vi "Drive_Heading.vi"(1 "Timeout (ms)":dbl, 2 "Speed (%)":dbl, 3 "Acceptable Error (in)":dbl, 4 "Distance (in)":dbl) -> (0 "Error (in)":dbl)   [LabVIEW 2020]
uses:
  <vilib>/Rock Robotics/WPI/ThirdParty/REV Robotics/REVLib/Typedef/Spark MAX Control Type.ctl
  <vilib>/Rock Robotics/WPI/ThirdParty/Phoenix-LabVIEW/Pigeon IMU/CTRE_PigeonIMU_GetYPR.vi
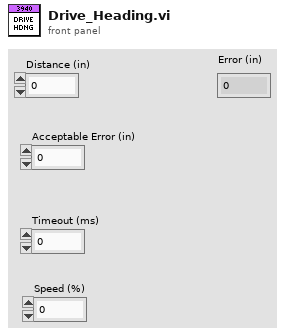
[diagram p1: front panel]
types:
  T1 = typedef "Spark MAX Control Type.ctl" = enum16{"Percent VBus", "Voltage", "Velocity", "Position", "Smart Motion", "Current", "Smart Velocity"}
  T2 = typedef "WPI_MotorControlDeviceRef.ctl" = cluster{"DeviceStatus":errorcluster, "Type":T3, "PWM":cluster{"PWM Channel":T4, "DeadBand":T5}, "CAN":cluster{"Device Number":u8, "SetOutput VI Ref":variant, "GetOutput VI Ref":variant, "Enable VI Ref":variant, "Disable VI Ref":variant, "Data":variant}, "Invert":bool, "DIO PWM":cluster{"PWM \"Enable\" Channel":T4, "DIOChannel":T6, "PWM Rate":dbl}}
  T3 = typedef "WPI_MotorControlType.ctl" = enum16{"PWM", "CAN", "DIO PWM"}
  T4 = typedef "FPGA_DIOPWMChannel.ctl" = enum8{"PWM 0", "PWM 1", "PWM 2", "PWM 3", "PWM 4", "PWM 5", "PWM 6", "PWM 7", "PWM 8", "PWM 9", "PWM MXP 0", "PWM MXP 1", "PWM MXP 2", "PWM MXP 3", "PWM MXP 4", "PWM MXP 5", "PWM MXP 6", "PWM MXP 7", "PWM MXP 8", "PWM MXP 9", "Invalid"}
  T5 = typedef "WPI_PWMDeadband.ctl" = cluster{"Name":string, "maxPositivePwm":i32, "minPositivePwm":i32, "centerPwm":i32, "maxNegativePwm":i32, "minNegativePwm":i32, "angularRange":u16}
  T6 = typedef "FPGA_DIOChannel.ctl" = enum8{"DIO 0", "DIO 1", "DIO 2", "DIO 3", "DIO 4", "DIO 5", "DIO 6", "DIO 7", "DIO 8", "DIO 9", "DIO MXP 0", "DIO MXP 1", "DIO MXP 2", "DIO MXP 3", "DIO MXP 4", "DIO MXP 5", "DIO MXP 6", "DIO MXP 7", "DIO MXP 8", "DIO MXP 9", "DIO MXP 10", "DIO MXP 11", "DIO MXP 12", "DIO MXP 13", "DIO MXP 14", "DIO MXP 15", "SPI Port CS1", "SPI Port CS2", "SPI Port CS3", "SPI Port MISO", "SPI Port MOSI", "Invalid"}
  T7 = typedef "CTRE_PigeonIMU_DeviceRef.ctl" = cluster{"DeviceStatus":errorcluster, "Device Number":u8, "Type":T8, "Device ID":u32, "Handle":u64, "UsageFrame":u32, "Library Path":path}
  T8 = typedef "CTRE_PigeonIMU_ConnectionType.ctl" = u32
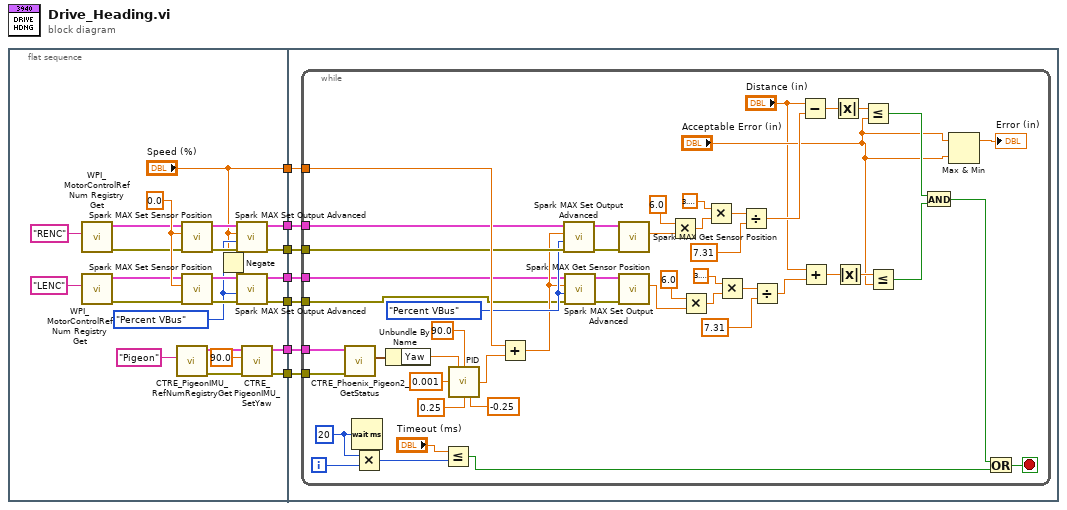
[diagram p0: block diagram]
diagram:
  n1 = flat-sequence {
    tunnel: [w23] -> w7
    tunnel: [w22] -> w6
    tunnel: [w21] -> w5
    tunnel: [w20] -> w4
    tunnel: [w10] -> w3
    tunnel: [w9] -> w2
    tunnel: ["Speed (%)"] -> w1
    tunnel: w7 -> [w38]
    tunnel: w6 -> [w37]
    tunnel: w5 -> [w36]
    tunnel: w4 -> [w35]
    tunnel: w3 -> [w34]
    tunnel: w2 -> [w33]
    tunnel: w1 -> [w32]
    frame #0 {
      w24 = Spark_MAX_Control_Type."Percent VBus" ("Control Mode")
      w25 = 0.0 ("Position")
      n2 = call <vilib>:"WPI_MotorControlRefNum Registry Get.vi"("refnum name"="RENC") -> ("error out"=w17:errorcluster, "MotorControlDevRef"=w18:T2)  [unwired: 9 in]
      n3 = call <vilib>:"WPI_MotorControlRefNum Registry Get.vi"("refnum name"="LENC") -> ("error out"=w15:errorcluster, "MotorControlDevRef"=w16:T2)  [unwired: 9 in]
      n4 = call <vilib>:"CTRE_PigeonIMU_RefNumRegistryGet.vi"("refnum name"="Pigeon") -> ("error out"=w14:errorcluster, "PigeonIMUDevRef"=w13:T7)  [unwired: 9 in]
      n5 = call <vilib>:"Spark MAX Set Sensor Position.vi"("error in"=w17, "Position"=w25, "MotorControlDeviceRef"=w18) -> ("error out"=w29:errorcluster, "MotorControlDeviceRef"=w28:T2)  [unwired: 7 in]
      n6 = call <vilib>:"Spark MAX Set Sensor Position.vi"("error in"=w15, "Position"=w25, "MotorControlDeviceRef"=w16) -> ("error out"=w27:errorcluster, "MotorControlDeviceRef"=w26:T2)  [unwired: 7 in]
      n7 = Negate(x="Speed (%)") -> (-x=w19:dbl)
      n8 = call <vilib>:"Spark MAX Set Output Advanced.vi"("error in (no error)"=w29, "Control Mode"=w24, "Setpoint"="Speed (%)", "MotorControlDevRef"=w28) -> ("error out"=w20:errorcluster, "MotorControlDevRef"=w23:T2)  [unwired: 6 in]
      n9 = call <vilib>:"Spark MAX Set Output Advanced.vi"("error in (no error)"=w27, "Control Mode"=w24, "Setpoint"=w19, "MotorControlDevRef"=w26) -> ("error out"=w21:errorcluster, "MotorControlDevRef"=w22:T2)  [unwired: 6 in]
      n10 = call <vilib>:"CTRE_PigeonIMU_SetYaw.vi"("error in (no error)"=w14, "Value"=90.0, "PigeonIMUDevRef"=w13) -> ("error out"=w9:errorcluster, "PigeonIMUDevRef"=w10:T7)  [unwired: 7 in]
    }
    frame #1 {
      n11 = while {
        tunnel: w38 -> [w47]
        tunnel: w37 -> [w41]
        tunnel: w36 -> [w40]
        tunnel: w35 -> [w46]
        tunnel: w34 -> [w58]
        tunnel: w33 -> [w57]
        tunnel: w32 -> [w48]
        i -> [w68]
        stop <- w62 stop-if-true
        w43 = Spark_MAX_Control_Type."Percent VBus" ("Control Mode")
        w67 = u32 20 ("milliseconds to wait")
        n12 = call-poly <vilib>:"CTRE_Phoenix_Pigeon2_GetStatus.vi"("error in (no error)"=w57, "PigeonIMUDevRef"=w58) -> ("Yaw Pitch Roll"=w59:cluster{"Yaw":dbl, "Pitch":dbl, "Roll":dbl})  [unwired: 7 in, 2 out]
        n13 = Wait (ms)(milliseconds to wait=w67) -> ()  [unwired: 1 out]
        n14 = Multiply(x=w67, y=w68) -> (x*y=w66:u32)
        n15 = Unbundle By Name(w59) -> ("Yaw"=w55:dbl)
        n16 = Less Or Equal?(x="Timeout (ms)", y=w66) -> (x <= y?=w64:bool)
        n17 = call "PID.vi"("Kp"=0.001, "Process Variable"=w55, "Goal"=90.0, "Max Ouput"=0.25, "Min Output"=-0.25) -> ("Command"=w49:dbl)  [unwired: 8 in, 2 out]
        n18 = Add(x=w48, y=w49) -> (x+y=w42:dbl)
        n19 = call <vilib>:"Spark MAX Set Output Advanced.vi"("error in (no error)"=w46, "Control Mode"=w43, "Setpoint"=w42, "MotorControlDevRef"=w47) -> ("error out"=w50:errorcluster, "MotorControlDevRef"=w51:T2)  [unwired: 6 in]
        n20 = call <vilib>:"Spark MAX Set Output Advanced.vi"("error in (no error)"=w40, "Control Mode"=w43, "Setpoint"=w42, "MotorControlDevRef"=w41) -> ("error out"=w44:errorcluster, "MotorControlDevRef"=w45:T2)  [unwired: 6 in]
        n21 = call <vilib>:"Spark MAX Get Sensor Position.vi"("error in (no error)"=w50, "MotorControlDevRef in"=w51) -> ("Sensor Position"=w88:dbl)  [unwired: 6 in, 3 out]
        n22 = call <vilib>:"Spark MAX Get Sensor Position.vi"("error in (no error)"=w44, "MotorControlDevRef in"=w45) -> ("Sensor Position"=w74:dbl)  [unwired: 6 in, 3 out]
        n23 = Multiply(x=6.0, y=w88) -> (x*y=w86:dbl)
        n24 = Multiply(x=6.0, y=w74) -> (x*y=w78:dbl)
        n25 = Multiply(x=3.141592653589793, y=w86) -> (x*y=w84:dbl)
        n26 = Multiply(x=3.141592653589793, y=w78) -> (x*y=w76:dbl)
        n27 = Divide(x=w84, y=7.31) -> (x/y=w82:dbl)
        n28 = Divide(x=w76, y=7.31) -> (x/y=w73:dbl)
        n29 = Subtract(x="Distance (in)", y=w82) -> (x-y=w81:dbl)
        n30 = Add(x="Distance (in)", y=w73) -> (x+y=w72:dbl)
        n31 = Absolute Value(x=w81) -> (abs(x)=w80:dbl)
        n32 = Absolute Value(x=w72) -> (abs(x)=w71:dbl)
        n33 = Less Or Equal?(x=w80, y="Acceptable Error (in)") -> (x <= y?=w70:bool)
        n34 = Less Or Equal?(x=w71, y="Acceptable Error (in)") -> (x <= y?=w69:bool)
        n35 = And(x=w70, y=w69) -> (x .and. y?=w63:bool)
        n36 = Max & Min(x="Acceptable Error (in)", y="Acceptable Error (in)") -> (max(x,y)=→"Error (in)":dbl)  [unwired: 1 out]
        n37 = Or(x=w63, y=w64) -> (x .or. y?=w62:bool)
      }
    }
  }
